vi "con^2 move all.vi"(8 "error in (no error)":errorcluster, 9 "now position":cluster{"x":dbl, "y":dbl, "degree":dbl}, 11 "contrast move array":T1[](array[typedef])) -> (0 "error out":errorcluster, 1 "position out":cluster{"x":dbl, "y":dbl, "degree":dbl})   [LabVIEW 2019]
uses:
  ctl/continued move array-V2.ctl
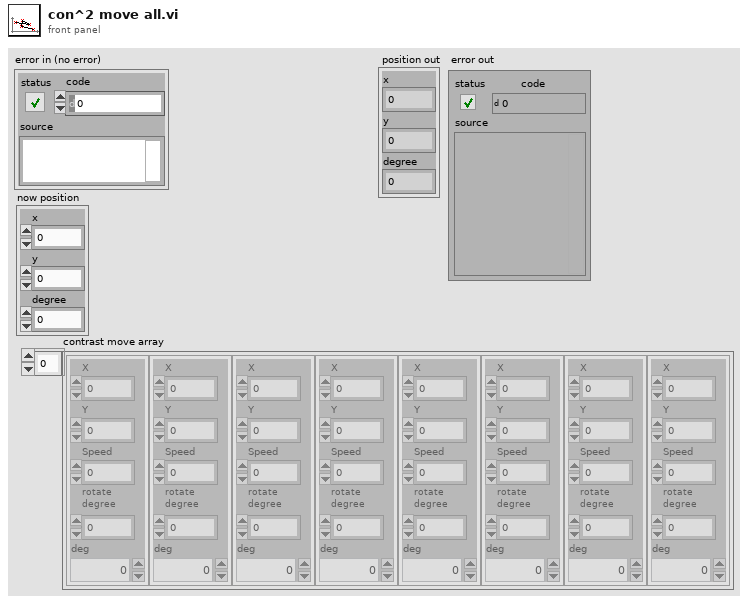
[diagram p1: front panel]
types:
  T1 = typedef "continued move array-V2.ctl" = cluster{"X":dbl, "Y":dbl, "Speed":dbl, "rotate\ndegree":dbl, "deg":dbl}
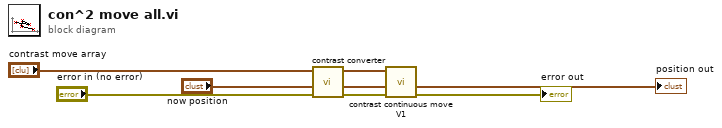
[diagram p0: block diagram]
diagram:
  n1 = call "contrast converter.vi"("now position"="now position", "contrast move array"="contrast move array") -> ("position out"=→"position out":cluster{"x":dbl, "y":dbl, "degree":dbl}, "move array"=w6:T1[])  [unwired: 8 in]
  n2 = call "contrast continuous move V1.vi"("error in (no error)"="error in (no error)", 11:w6) -> ("error out"=→"error out":errorcluster)  [unwired: 9 in]
